vi "Close Data File and open.vi"(8 "error in":errorcluster, 11 "File Refnum In":refnum<file>) -> (0 "error out":errorcluster, 3 "path":path)   [LabVIEW 2018]
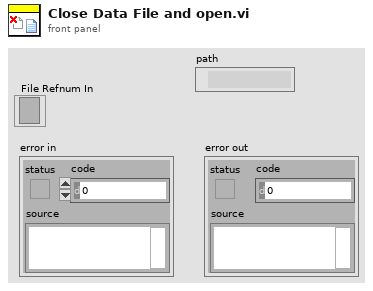
[diagram p1: front panel]
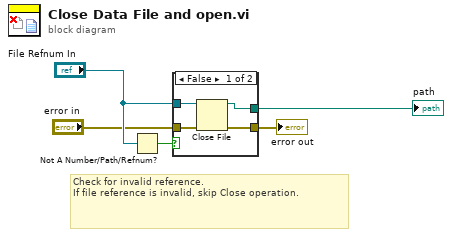
[diagram p0: block diagram]
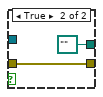
[diagram p2: hidden frame]
diagram:
  # "Check for invalid reference. \nIf file reference is invalid, skip Close operation."
  n1 = Not A Number/Path/Refnum?(number/path/refnum="File Refnum In") -> (NaN/Path/Refnum?=w5:bool)
  n2 = case shown="False" w5 {
    tunnel: "error in" -> [w9 w11]
    tunnel: "File Refnum In" -> [w8 _]
    tunnel: [w7 w11] -> w3
    tunnel: [w6 path "" ("path")] -> w1
    frame False {
      n3 = Close File(refnum=w8, error in=w9) -> (path=w6:path, error out=w7:errorcluster)
    }
    frame True {
    }
  }
  "error out" <- w3
  "path" <- w1
